vi "Read Remote Port.vi"(11 "TCP Stream in":refnum<class "TCP Stream.lvclass">) -> (2 "remote port":u16=2001)   [LabVIEW 2020, in "TCP Stream.lvclass"]
doc: "Returns the IP port of the remote connection."
uses:
  TCP Stream.lvclass
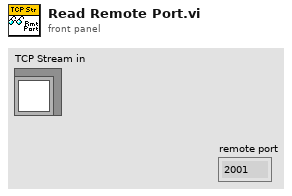
[diagram p1: front panel]
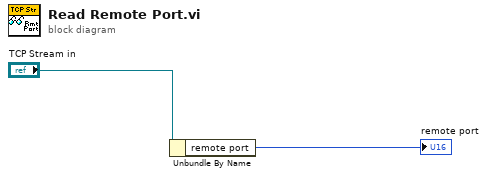
[diagram p0: block diagram]
diagram:
  n1 = Unbundle By Name("TCP Stream in") -> ("remote port"=→"remote port":u16)
